vi "ExtractRouterInfo.vi"(1 "router channel":u16, 2 "Array 2":u32[][][][](array[numeric])) -> (0 "Array":u32[][][][](array[numeric]))   [LabVIEW 2009]
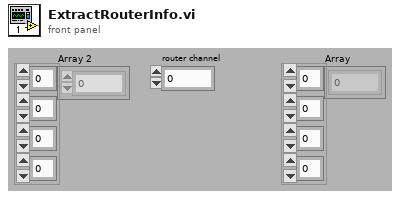
[diagram p1: front panel]
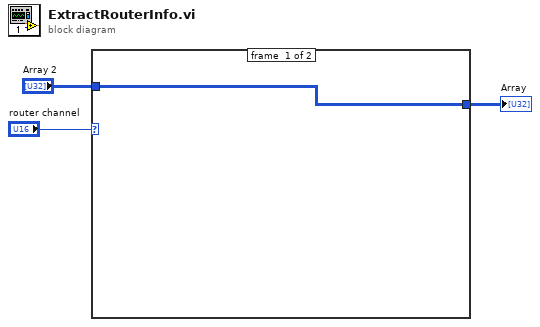
[diagram p0: block diagram]
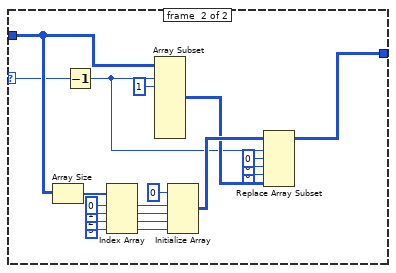
[diagram p2: hidden frame]
diagram:
  n1 = case shown="0, Default" "router channel" {
    selector: "router channel" -> [_ w12]
    tunnel: "Array 2" -> [w4 w23]
    tunnel: [w4 w10] -> w1
    frame #0 {
    }
    frame #1 {
      n2 = Array Size(array=w23) -> (size(s)=w22:i32[])
      n3 = Decrement(x=w12) -> (x-1=w5:u16)
      n4 = Index Array(array=w22, index #1=0 ("index"), index #2=1 ("index"), index #3=2 ("index"), index #4=3 ("index")) -> (element #1=w16:i32, element #2=w15:i32, element #3=w14:i32, element #4=w13:i32)
      n5 = Array Subset(array=w23, index (dim 0)=w5, length (dim 0)=1 ("length")) -> (w6:u32[][][][])  [unwired: 6 in]
      n6 = Initialize Array(u32 0 ("element"), w16, w15, w14, w13) -> (w11:u32[][][][])
      n7 = Replace Array Subset(array=w11, new element=w6, index (dim 0)=w5, index (dim 1)=0 ("disabled index (page)"), index (dim 2)=0 ("disabled index (row)"), index (dim 3)=0 ("disabled index (col)")) -> (w10:u32[][][][])
    }
  }
  "Array" <- w1
